vi "Porównanie.vi"(1 "porownanie":i32[][](array[numeric]), 2 "miny":i32[][](array[numeric]), 3 "Rozmiar":i32) -> (0 "Array":i32[][](array[numeric]))   [LabVIEW 2021]
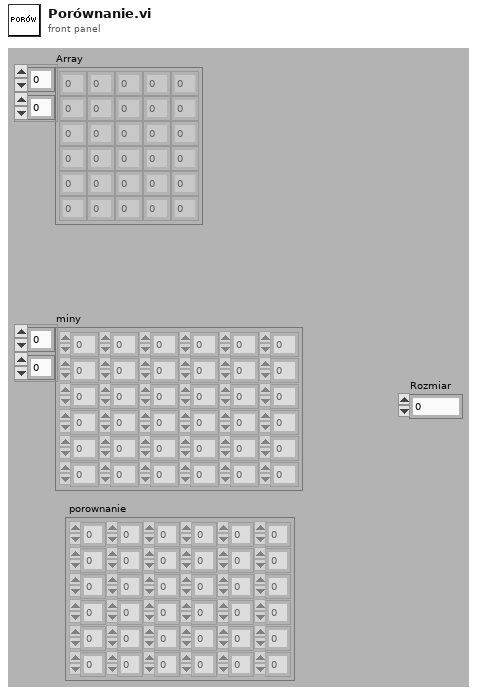
[diagram p1: front panel]
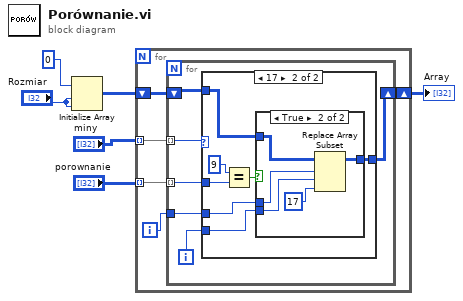
[diagram p0: block diagram]
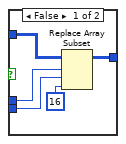
[diagram p3: hidden frame]
diagram:
  n1 = Initialize Array(0 ("element"), "Rozmiar", "Rozmiar") -> (w4:i32[][])
  n2 = for {
    tunnel: "porownanie" -> [w11] mode=indexing
    shift-right: [w9] -> w1
    shift-left: w4 -> [w8]
    tunnel: "miny" -> [w7] mode=indexing
    i -> [w10]
    n3 = for {
      tunnel: w11 -> [w17] mode=indexing
      tunnel: w10 -> [w16]
      shift-right: [w14] -> w9
      shift-left: w8 -> [w15]
      tunnel: w7 -> [w12] mode=indexing
      i -> [w13]
      n4 = case shown="17" w12 {
        tunnel: w13 -> [_ w22]
        tunnel: w17 -> [_ w25]
        tunnel: w16 -> [_ w21]
        tunnel: w15 -> [w18 w20]
        tunnel: [w18 w19] -> w14
        frame 0, Default {
        }
        frame 17 {
          n5 = Equal?(x=9 ("CONTADOR"), y=w25) -> (x = y?=w23:bool)
          n6 = case shown="True" w23 {
            tunnel: w20 -> [w26 w31]
            tunnel: [w29 w35] -> w19
            tunnel: w22 -> [w27 w33]
            tunnel: w21 -> [w28 w32]
            frame False {
              n7 = Replace Array Subset(array=w26, new element=16 ("new element/subarray"), index (row)=w28, index (col)=w27) -> (w29:i32[][])
            }
            frame True {
              n8 = Replace Array Subset(array=w31, new element=17 ("CONTADOR"), index (row)=w32, index (col)=w33) -> (w35:i32[][])
            }
          }
        }
      }
    }
  }
  "Array" <- w1
